vi "New Vision Server.vi"(2 "error in":errorcluster, 3 "TCP Port":u16) -> (0 "error out":errorcluster, 1 "Vision Server":T1)   [LabVIEW 2016]
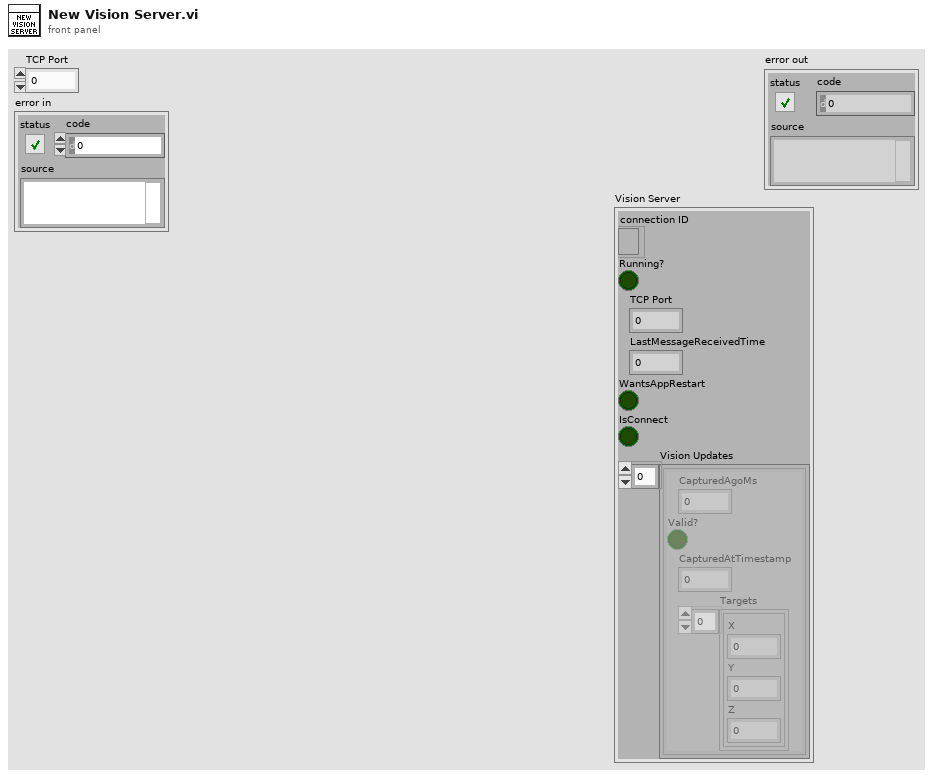
[diagram p1: front panel]
types:
  T1 = cluster{"connection ID":refnum<k5>, "Running?":bool, "TCP Port":u16, "LastMessageReceivedTime":dbl, "WantsAppRestart":bool, "IsConnect":bool, "Vision Updates":cluster{"CapturedAgoMs":i32, "Valid?":bool, "CapturedAtTimestamp":dbl, "Targets":cluster{"X":dbl, "Y":dbl, "Z":dbl}[]}[]}
  T2 = cluster{"CapturedAgoMs":i32, "Valid?":bool, "CapturedAtTimestamp":dbl, "Targets":cluster{"X":dbl, "Y":dbl, "Z":dbl}[]}[]
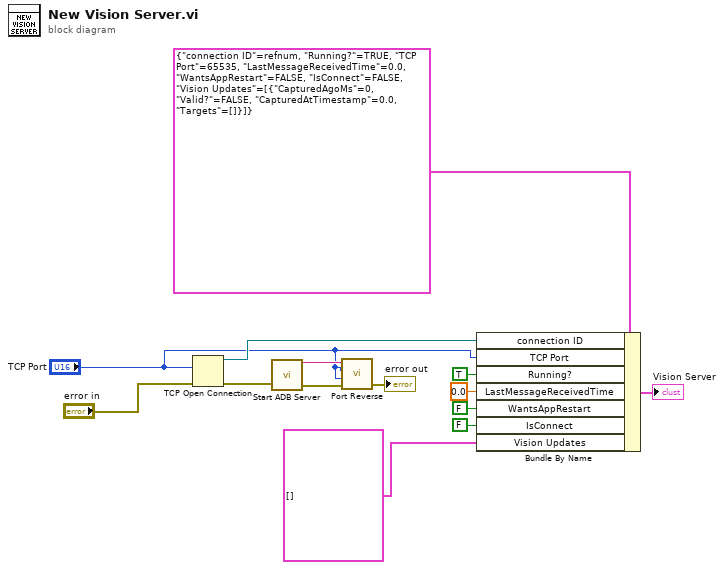
[diagram p0: block diagram]
diagram:
  n1 = TCP Open Connection(remote port or service name="TCP Port", error in (no error)="error in") -> (connection ID=w8:refnum<k5>, error out=w13:errorcluster)  [unwired: 3 in]
  n2 = call "Start ADB Server.vi"("error in"=w13) -> ("standard output"=w12:string, "error out"=w11:errorcluster)  [unwired: 1 in, 1 out]
  n3 = call "Port Reverse.vi"("error in"=w11, "local TCP port"="TCP Port", "remote TCP port"="TCP Port", "adb location"=w12) -> ("error out"=→"error out":errorcluster)  [unwired: 2 out]
  n4 = Bundle By Name(cluster=T1 {"connection ID"=refnum, "Running?"=TRUE, "TCP Port"=65535, "LastMessageReceivedTime"=0.0, "WantsAppRestart"=FALSE, "IsConnect"=FALSE, "Vision Updates"=[{"CapturedAgoMs"=0, "Valid?"=FALSE, "CapturedAtTimestamp"=0.0, "Targets"=[]}]}, "connection ID"=w8, "TCP Port"="TCP Port", "Running?"=TRUE, "LastMessageReceivedTime"=0.0, "WantsAppRestart"=FALSE, "IsConnect"=FALSE, "Vision Updates"=T2 []) -> (→"Vision Server":T1)
